vi "CHD_DRIVE_Get_SpeedDmd.vi"() -> (1 "RightSpeedDmd_MpserS":dbl, 3 "LeftSpeedDmd_MperS":dbl, 4 "MotorSpeedDmds_MperSec":dbl[](array[numeric]) format="%17.2f")   [LabVIEW 2019]
uses:
  CHD_DRIVE_GLOBALS.vi
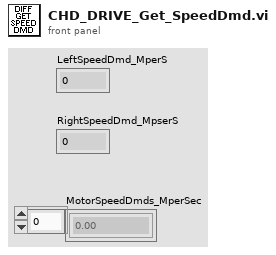
[diagram p1: front panel]
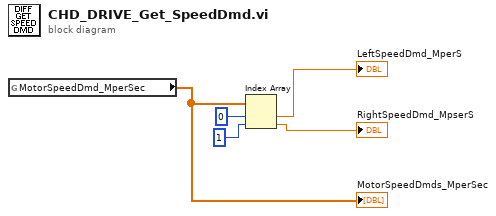
[diagram p0: block diagram]
diagram:
  n1 = global read "CHD_DRIVE_GLOBALS.vi" "MotorSpeedDmd_MperSec"() -> (w3:dbl[])
  "MotorSpeedDmds_MperSec" <- w3
  n2 = Index Array(array=w3, index #1=0 ("index"), index #2=1 ("index")) -> (element #1=→"LeftSpeedDmd_MperS":dbl, element #2=→"RightSpeedDmd_MpserS":dbl)
